vi "Check Win Lose.vi"(8 "error in (no error)":errorcluster, 11 "Game Data in":T1) -> (0 "error out":errorcluster, 1 "Lose?":bool, 2 "Win?":bool, 3 "Game Data out":T1)   [LabVIEW 2025]
uses:
  Game Data.ctl
  Bullet Data.ctl
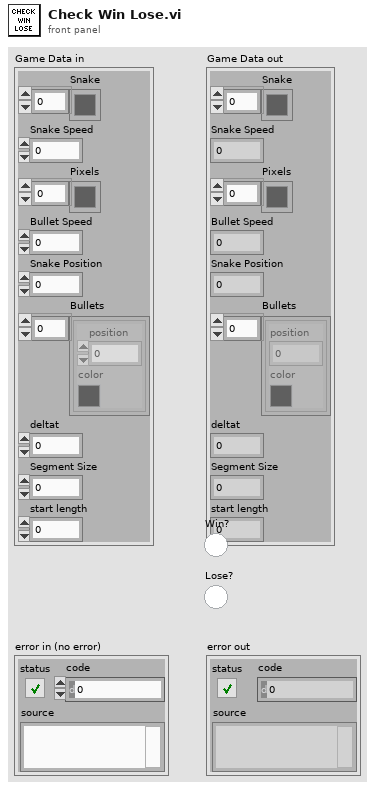
[diagram p1: front panel]
types:
  T1 = typedef "Game Data.ctl" = cluster{"Snake":u32[], "Snake Speed":dbl, "Pixels":u32[], "Bullet Speed":dbl, "Snake Position":dbl, "Bullets":T2[], "deltat":dbl, "Segment Size":dbl, "start length":u32}
  T2 = typedef "Bullet Data.ctl" = cluster{"position":dbl, "color":u32}
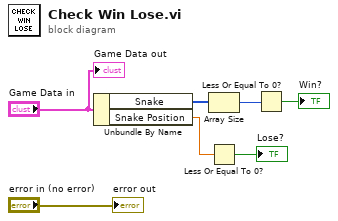
[diagram p0: block diagram]
diagram:
  n1 = Unbundle By Name("Game Data in") -> ("Snake"=w5:u32[], "Snake Position"=w2:dbl)
  n2 = Array Size(array=w5) -> (size(s)=w4:i32)
  n3 = Less Or Equal To 0?(x=w2) -> (x <= 0?=→"Lose?":bool)
  n4 = Less Or Equal To 0?(x=w4) -> (x <= 0?=→"Win?":bool)
  "error out" <- "error in (no error)"
  "Game Data out" <- "Game Data in"
